vi "CMN_toGUIDE.vi"(7 "pointer":u64, 8 "error in (no error)":errorcluster, 9 "ms timeout (-1)":i32=-1, 10 "responseQ":string, 11 "Command":string) -> (0 "error out":errorcluster, 2 "response":string)   [LabVIEW 2016]
panel:
  in  "SGUIDE struct":T1
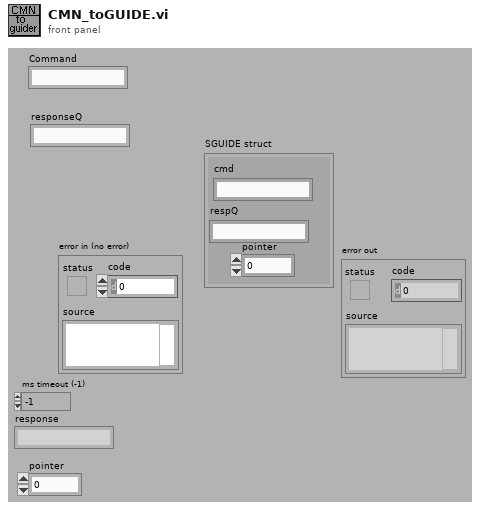
[diagram p1: front panel]
types:
  T1 = cluster{"cmd":string, "respQ":string, "pointer":u64}
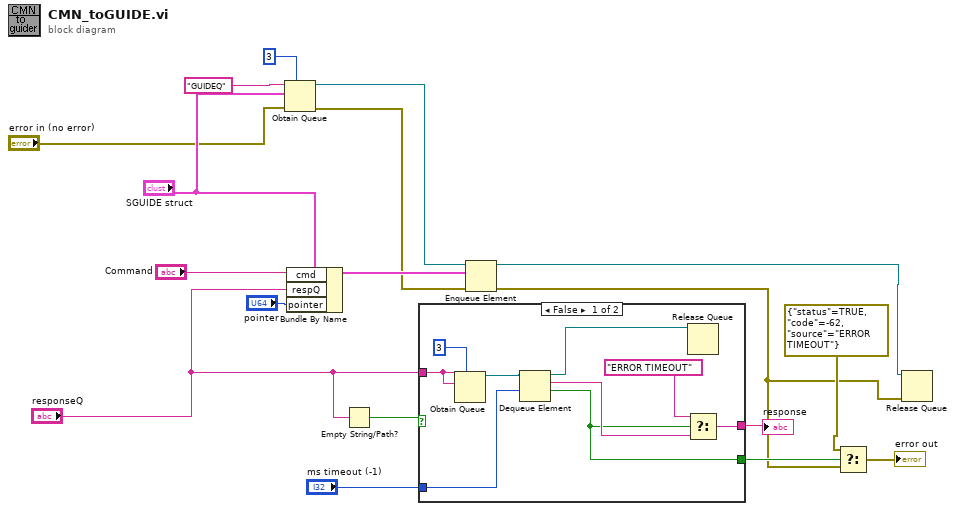
[diagram p0: block diagram]
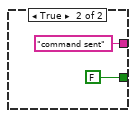
[diagram p2: hidden frame]
diagram:
  n1 = Obtain Queue(max queue size (-1, unlimited)=3, name (unnamed)="GUIDEQ", element data type="SGUIDE struct", error in (no error)="error in (no error)") -> (queue out=w16:refnum<queue>, error out=w8:errorcluster)  [unwired: 1 in, 1 out]
  n2 = Bundle By Name(cluster="SGUIDE struct", "cmd"="Command", "respQ"="responseQ", "pointer"="pointer") -> (w14:T1)
  n3 = Empty String/Path?(string/path="responseQ") -> (empty?=w12:bool)
  n4 = case shown="False" w12 {
    tunnel: "responseQ" -> [w27 _]
    tunnel: "ms timeout (-1)" -> [w25 _]
    tunnel: [w22 "command sent"] -> w10
    tunnel: [w21 FALSE ("timed out?")] -> w7
    frame False {
      n5 = Obtain Queue(max queue size (-1, unlimited)=3, name (unnamed)=w27, element data type=w27) -> (queue out=w26:refnum<queue>)  [unwired: 2 in, 2 out]
      n6 = Dequeue Element(queue=w26, timeout in ms (-1)=w25) -> (queue out=w20:refnum<queue>, element=w24:string, timed out?=w21:bool)  [unwired: 1 in, 1 out]
      n7 = Release Queue(queue=w20) -> ()  [unwired: 1 in, 4 out]
      n8 = Select(t="ERROR TIMEOUT", s=w21, f=w24) -> (s? t:f=w22:string)
    }
    frame True {
    }
  }
  "response" <- w10
  n9 = Enqueue Element(queue=w16, element=w14, error in (no error)=w8) -> (queue out=w3:refnum<queue>, error out=w2:errorcluster)  [unwired: 2 out]
  n10 = Select(t=errorcluster {"status"=TRUE, "code"=-62, "source"="ERROR TIMEOUT"}, s=w7, f=w2) -> (s? t:f=→"error out":errorcluster)
  n11 = Release Queue(queue=w3, error in (no error)=w2) -> ()  [unwired: 4 out]
